vi "RemoveNaN(1D).vi"() -> ()   [LabVIEW 2010]
panel:
  out "Exec Time (ms)":u32
  out "length":i32
  out "Array Out":sgl[](array[numeric]) format="%.3f"
  in  "Array IN":sgl[](array[numeric]) format="%.3f"
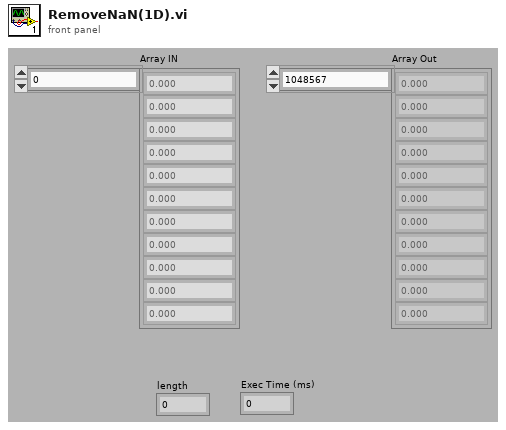
[diagram p1: front panel]
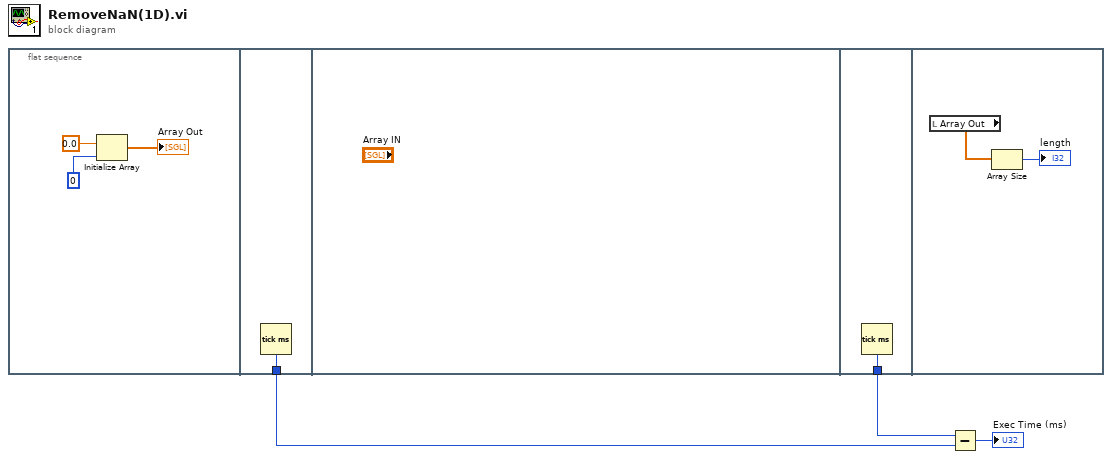
[diagram p0: block diagram]
diagram:
  n1 = flat-sequence {
    tunnel: [w7] -> w2
    tunnel: [w8] -> w3
    frame #0 {
      n2 = Initialize Array(sgl 0.0 ("element"), 0 ("dimension size")) -> (→"Array Out":sgl[])
    }
    frame #1 {
      n3 = Tick Count (ms)() -> (millisecond timer value=w7:u32)
    }
    frame #2 {
    }
    frame #3 {
      n4 = Tick Count (ms)() -> (millisecond timer value=w8:u32)
    }
    frame #4 {
      n5 = local read "Array Out"() -> (w10:sgl[])
      n6 = Array Size(array=w10) -> (size(s)=→"length":i32)
    }
  }
  n7 = Subtract(x=w3, y=w2) -> (x-y=→"Exec Time (ms)":u32)
